vi "Decode Operator Packet.vi"(10 "Type ID":u32, 11 "Bit Stream in":bool[](array[boolean])) -> (0 "Length Type ID":u32, 1 "Value":u64, 2 "Packets Out":T1[](array[typedef]), 3 "Bit Stream out":bool[](array[boolean]))   [LabVIEW 2019, in "Day 16.lvlib"]
uses:
  Day 16.lvlib
  Controls/Packet.ctl
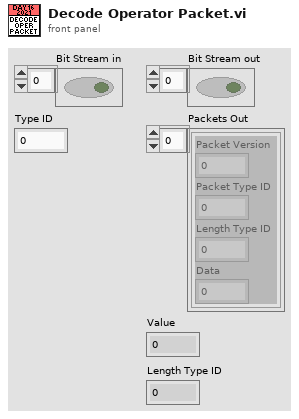
[diagram p1: front panel]
types:
  T1 = typedef "Day 16.lvlib/Packet.ctl" = cluster{"Packet Version":u32, "Packet Type ID":u32, "Length Type ID":u32, "Data":u64}
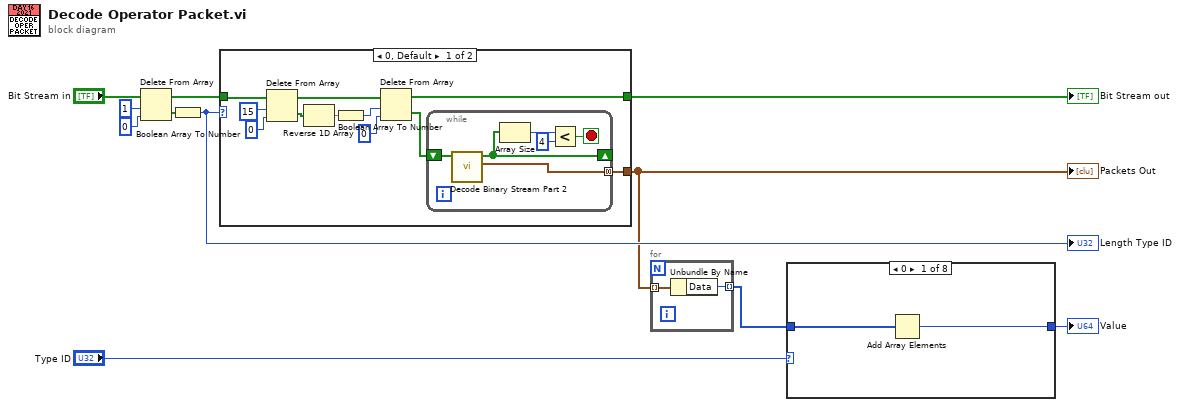
[diagram p0: block diagram]
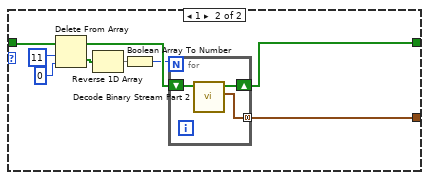
[diagram p2: hidden frame]
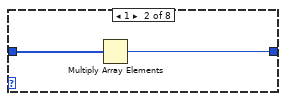
[diagram p3: hidden frame]
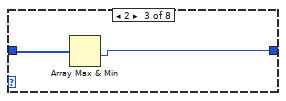
[diagram p4: hidden frame]
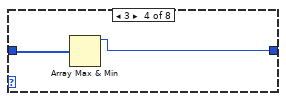
[diagram p5: hidden frame]
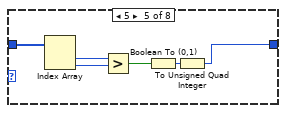
[diagram p6: hidden frame]
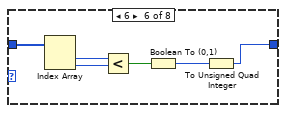
[diagram p7: hidden frame]
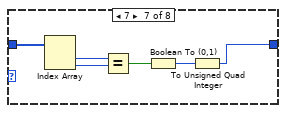
[diagram p8: hidden frame]
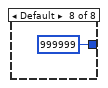
[diagram p9: hidden frame]
diagram:
  n1 = Delete From Array(array="Bit Stream in", length=1, index=0) -> (deleted portion=w8:bool[], array with subset deleted=w10:bool[])
  n2 = Boolean Array To Number(Boolean array=w8) -> (number=w9:u32)
  "Length Type ID" <- w9
  n3 = case shown="0, Default" w9 {
    tunnel: w10 -> [w20 w35]
    tunnel: [w14 w29] -> w11
    tunnel: [w12 w32] -> w3
    frame 0, Default {
      n4 = Delete From Array(array=w20, length=15, index=0) -> (deleted portion=w17:bool[], array with subset deleted=w15:bool[])
      n5 = Reverse 1D Array(array=w17) -> (reversed array=w18:bool[])
      n6 = Boolean Array To Number(Boolean array=w18) -> (number=w16:u32)
      n7 = Delete From Array(array=w15, length=w16, index=0) -> (deleted portion=w13:bool[], array with subset deleted=w14:bool[])
      n8 = while {
        tunnel: [w27] -> w12 mode=concatenating
        shift-right: [w23] -> _
        shift-left: w13 -> [w28]
        stop <- w24 stop-if-true
        n9 = call "Decode Binary Stream Part 2.vi"("Bit Stream"=w28) -> ("Packets Out"=w27:T1[], "Bit Stream Out"=w23:bool[])  [unwired: 9 in]
        n10 = Array Size(array=w23) -> (size(s)=w26:i32)
        n11 = Less?(x=w26, y=4) -> (x < y?=w24:bool)
      }
    }
    frame 1 {
      n12 = Delete From Array(array=w35, length=11, index=0) -> (deleted portion=w33:bool[], array with subset deleted=w31:bool[])
      n13 = Reverse 1D Array(array=w33) -> (reversed array=w34:bool[])
      n14 = Boolean Array To Number(Boolean array=w34) -> (number=w30:u32)
      n15 = for {
        N: w30 -> [_]
        tunnel: [w39] -> w32 mode=concatenating
        shift-right: [w38] -> w29
        shift-left: w31 -> [w40]
        n16 = call "Decode Binary Stream Part 2.vi"("Bit Stream"=w40) -> ("Packets Out"=w39:T1[], "Bit Stream Out"=w38:bool[])  [unwired: 9 in]
      }
    }
  }
  "Packets Out" <- w3
  "Bit Stream out" <- w11
  n17 = for {
    tunnel: w3 -> [w42] mode=indexing
    tunnel: [w41] -> w2 mode=indexing
    n18 = Unbundle By Name(w42) -> ("Data"=w41:u64)
  }
  n19 = case shown="0" "Type ID" {
    tunnel: w2 -> [w44 w46 w48 w50 w56 w62 w68 _]
    tunnel: [w43 w45 w47 w49 w51 w57 w63 u64 999999 ("Data")] -> w1
    frame 0 {
      n20 = Add Array Elements(numeric array=w44) -> (sum=w43:u64)
    }
    frame 1 {
      n21 = Multiply Array Elements(1:w46) -> (0:w45:u64)
    }
    frame 2 {
      n22 = Array Max & Min(array=w48) -> (min value=w47:u64)  [unwired: 3 out]
    }
    frame 3 {
      n23 = Array Max & Min(array=w50) -> (max value=w49:u64)  [unwired: 3 out]
    }
    frame 5 {
      n24 = Index Array(array=w56) -> (element #1=w55:u64, element #2=w54:u64)  [unwired: 2 in]
      n25 = Greater?(x=w55, y=w54) -> (0:w53:bool)
      n26 = Boolean To (0,1)(Boolean=w53) -> (0, 1=w52:i16)
      n27 = To Unsigned Quad Integer(1:w52) -> (0:w51:u64)
    }
    frame 6 {
      n28 = Index Array(array=w62) -> (element #1=w61:u64, element #2=w60:u64)  [unwired: 2 in]
      n29 = Less?(x=w61, y=w60) -> (x < y?=w59:bool)
      n30 = Boolean To (0,1)(Boolean=w59) -> (0, 1=w58:i16)
      n31 = To Unsigned Quad Integer(1:w58) -> (0:w57:u64)
    }
    frame 7 {
      n32 = Index Array(array=w68) -> (element #1=w67:u64, element #2=w66:u64)  [unwired: 2 in]
      n33 = Equal?(x=w67, y=w66) -> (x = y?=w65:bool)
      n34 = Boolean To (0,1)(Boolean=w65) -> (0, 1=w64:i16)
      n35 = To Unsigned Quad Integer(1:w64) -> (0:w63:u64)
    }
    frame Default {
    }
  }
  "Value" <- w1
